vi "Draw Border.vi"(8 "error in (no error)":errorcluster, 11 "Triangle in":refnum<class "Rectangle.lvclass">) -> (0 "error out":errorcluster, 2 "Picture out":picture, 3 "Triangle out":refnum<class "Rectangle.lvclass">)   [LabVIEW 2015, in "Rectangle.lvclass"]
uses:
  Rectangle.lvclass
  Rectangle Border/Rectangle Border.lvclass
  Graphic/Graphic.lvclass/Graphic.ctl
  Rectangle Border/Rectangle Border.lvclass/Rectangle Border.ctl
  Scalable Border/Scalable Border.lvclass
  Graphic/Graphic.lvclass
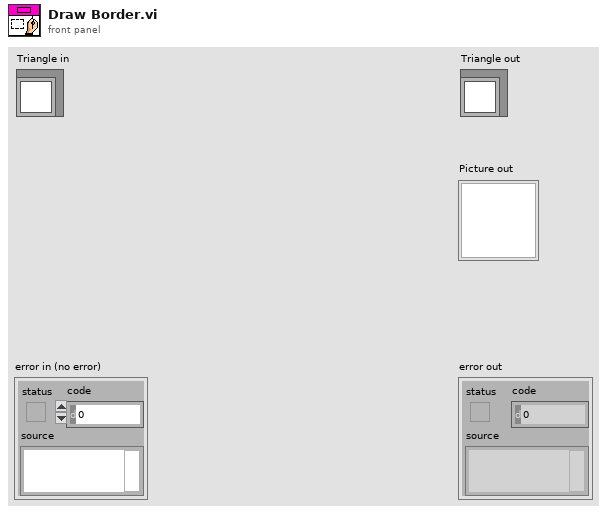
[diagram p1: front panel]
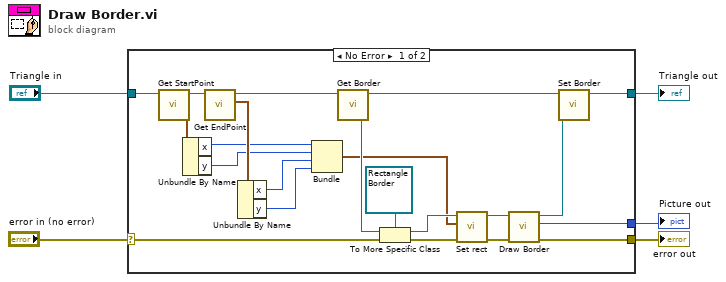
[diagram p0: block diagram]
diagram:
  n1 = case shown="No Error" "error in (no error)" {
    selector: "error in (no error)" -> [w10 w29]
    tunnel: "Triangle in" -> [w27 w28]
    tunnel: [w7 w28] -> w4
    tunnel: [w9 w29] -> w2
    tunnel: [w8 _] -> w1
    frame No Error {
      n2 = call "Get StartPoint.vi"("Graphic in"=w27) -> ("StartPoint"=w18:cluster{"x":i16, "y":i16}, "Graphic out"=w20:refnum<class "Rectangle.lvclass">)  [unwired: 8 in, 1 out]
      n3 = Unbundle By Name(w18) -> ("x"=w16:i16, "y"=w15:i16)
      n4 = call "Get EndPoint.vi"("Graphic in"=w20) -> ("EndPoint"=w17:cluster{"x":i16, "y":i16}, "Graphic out"=w19:refnum<class "Rectangle.lvclass">)  [unwired: 8 in, 1 out]
      n5 = Unbundle By Name(w17) -> ("x"=w14:i16, "y"=w13:i16)
      n6 = Bundle("x"=w16, "y"=w15, "x"=w14, "y"=w13) -> (w12:cluster{"x":i16, "y":i16, "x":i16, "y":i16})  [unwired: 1 in]
      n7 = call "Get Border.vi"("Graphic in"=w19) -> ("Scalable Border.lvclass"=w24:refnum<class "Scalable Border.lvclass">, "Graphic out"=w26:refnum<class "Rectangle.lvclass">)  [unwired: 8 in, 1 out]
      n8 = To More Specific Class(target class=refnum<class "Rectangle Border.lvclass"> refnum ("Rectangle Border.lvclass"), reference=w24, error in=w10) -> (specific class reference=w22:refnum<class "Rectangle Border.lvclass">, error out=w23:errorcluster)
      n9 = call "Set rect.vi"("error in (no error)"=w23, "rect"=w12, "Rectangle Border in"=w22) -> ("error out"=w11:errorcluster, "Rectangle Border out"=w25:refnum<class "Rectangle Border.lvclass">)  [unwired: 7 in]
      n10 = call-dynamic "Draw Border.vi"("error in (no error)"=w11, "Rectangle Border in"=w25) -> ("error out"=w9:errorcluster, "Border out"=w8:picture, "Rectangle Border out"=w6:refnum<class "Rectangle Border.lvclass">)  [unwired: 7 in]
      n11 = call "Set Border.vi"("Scalable Border.lvclass"=w6, "Graphic in"=w26) -> ("Graphic out"=w7:refnum<class "Rectangle.lvclass">)  [unwired: 8 in, 1 out]
    }
    frame Error {
    }
  }
  "error out" <- w2
  "Triangle out" <- w4
  "Picture out" <- w1
